vi "Global variables.vi"() -> ()   [LabVIEW 2014]
panel:
  in  "Average":i32=1
  in  "Integration Time":i32=100
  in  "Correct Electrical Dark":bool
  out "error IO":errorcluster
  out "VISA refnum":refnum<visa-resource-name>
  out "Number of Spectrometers":i32
  out "Wrapper":u32
  # "Spectrometer"
  # "Power Meter"
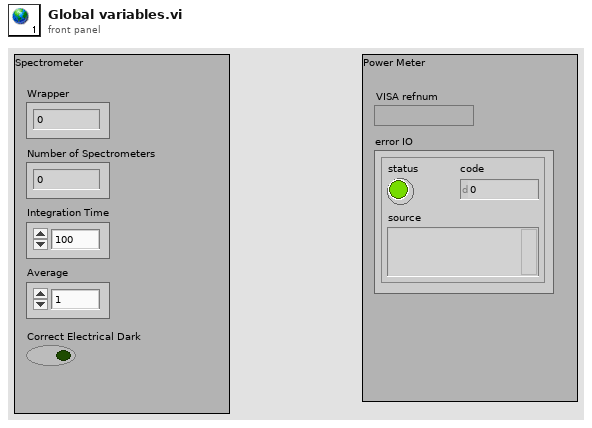
[diagram p1: front panel]
diagram:
